vi "FindRepeated (SubVI).vi"(1 "time stamp":dbl[](array[numeric])) -> (0 "not repeated?":bool[](array[boolean]))   [LabVIEW 2017]
uses:
  <vilib>/Analysis/NI_AALPro.lvlib
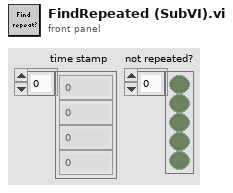
[diagram p1: front panel]
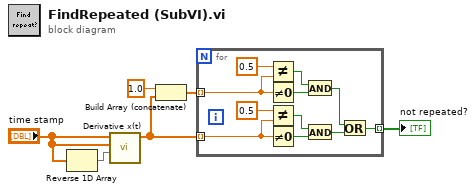
[diagram p0: block diagram]
diagram:
  n1 = Reverse 1D Array(array="time stamp") -> (reversed array=w3:dbl[])
  n2 = call <vilib>:"Derivative x(t).vi"("Final Condition"=w3, "Initial Condition"="time stamp", "X"="time stamp") -> ("dX/dt"=w2:dbl[])  [unwired: 7 in, 1 out]
  n3 = Build Array (concatenate)(1.0, w2) -> (w4:dbl[])
  n4 = for {
    tunnel: w4 -> [w11] mode=indexing
    tunnel: w2 -> [w8] mode=indexing
    tunnel: [w7] -> w6 mode=indexing
    n5 = Not Equal?(x=0.5, y=w11) -> (x != y?=w13:bool)
    n6 = Not Equal To 0?(x=w11) -> (x != 0?=w14:bool)
    n7 = Not Equal?(x=0.5, y=w8) -> (x != y?=w16:bool)
    n8 = Not Equal To 0?(x=w8) -> (x != 0?=w15:bool)
    n9 = And(x=w13, y=w14) -> (x .and. y?=w9:bool)
    n10 = And(x=w16, y=w15) -> (x .and. y?=w10:bool)
    n11 = Or(x=w9, y=w10) -> (x .or. y?=w7:bool)
  }
  "not repeated?" <- w6
